vi "Launch Reader.vi"(8 "error in (no error)":errorcluster, 11 "ConnectionManager in":refnum<class "ConnectionManager.lvclass">) -> (0 "error out":errorcluster, 3 "ConnectionManager out":refnum<class "ConnectionManager.lvclass">)   [LabVIEW 2020, in "ConnectionManager.lvlib" / "ConnectionManager.lvclass"]
uses:
  <vilib>/gpm_packages/@cs/Network-interface/Source/ConnectionManager/ConnectionManager/ConnectionManager.lvclass
  C:/Program Files/National Instruments/LabVIEW 2020/vi.lib/ActorFramework/Actor/Actor.lvclass
  C:/Program Files/National Instruments/LabVIEW 2020/vi.lib/gpm_packages/@cs/Network-interface/Source/Logged Actor/LoggedActor.lvclass
  <vilib>/gpm_packages/@cs/Network-interface/Source/Logged Actor/LoggedActor.lvclass/LoggedActor.ctl
  <vilib>/gpm_packages/@cs/Network-interface/Source/ConnectionManager/ConnectionManager/ConnectionManager.lvclass/ConnectionManager.ctl
  <vilib>/gpm_packages/@cs/Network-interface/Source/ConnectionReader/ConnectionReader/ConnectionReader.lvclass
  <vilib>/ActorFramework/Actor/Actor.lvclass
  <vilib>/gpm_packages/@cs/Network-interface/Source/Logged Actor/LoggedActor.lvclass
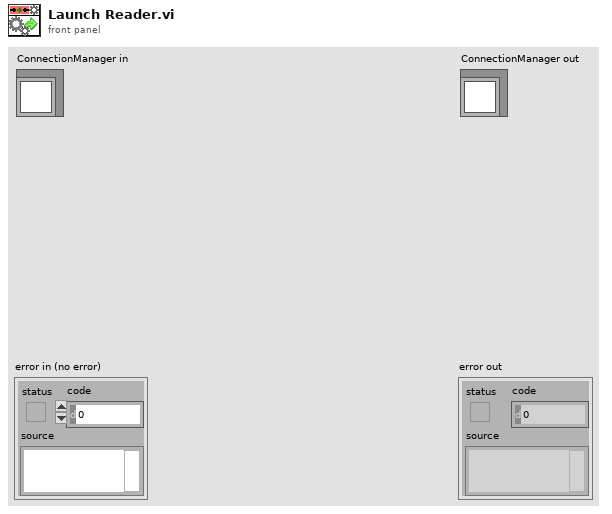
[diagram p1: front panel]
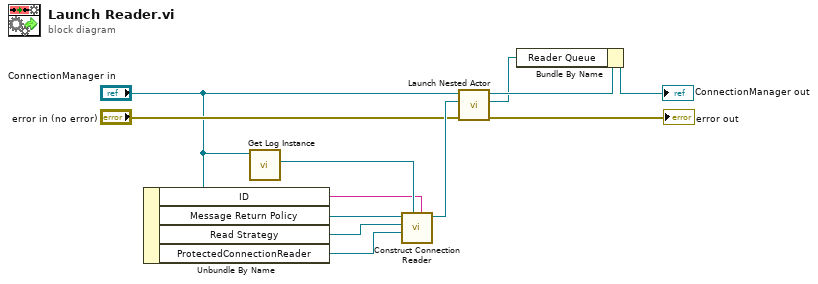
[diagram p0: block diagram]
diagram:
  n1 = Unbundle By Name("ConnectionManager in") -> ("ID"=w1:string, "Message Return Policy"=w8:refnum<class "IMessageReturnPolicy.lvclass">, "Read Strategy"=w7:refnum<class "IReadStrategy.lvclass">, "ProtectedConnectionReader"=w4:refnum<class "ProtectedConnectionReader.lvclass">)
  n2 = call <vilib>:"Get Log Instance.vi"("LoggedActor in"="ConnectionManager in") -> ("Log Instance"=w2:refnum<class "LoggerReference.lvclass">)  [unwired: 8 in, 2 out]
  n3 = call <vilib>:"Construct Connection Reader.vi"("Log Alias"=w1, "Log Instance"=w2, "ProtectedConnection"=w4, "ReadStrategy"=w7, "Message Return Policy"=w8) -> ("ConnectionReader out"=w12:refnum<class "ConnectionReader.lvclass">)  [unwired: 6 in]
  n4 = call <vilib>:"Launch Nested Actor.vi"("error in (no error)"="error in (no error)", "Nested Actor"=w12, "Caller Actor in"="ConnectionManager in") -> ("error out"=→"error out":errorcluster, "Nested Actor's Enqueuer"=w9:refnum<class "Message Enqueuer.lvclass">, "Caller Actor out"=w11:refnum<class "ConnectionManager.lvclass">)  [unwired: 6 in]
  n5 = Bundle By Name(cluster=w11, "Reader Queue"=w9) -> (→"ConnectionManager out":refnum<class "ConnectionManager.lvclass">)
